vi "Assert Selection.vi"(9 "Actual":T1, 10 "Expected":T1, 11 "Added Section Finder Test In":refnum<class "Added Section Finder Test.lvclass">) -> (0 "error out":errorcluster, 3 "Added Section Finder Test Out":refnum<class "Added Section Finder Test.lvclass">)   [LabVIEW 2020, in "Added Section Finder Test.lvclass"]
uses:
  Added Section Finder Test.lvclass
  usr/local/natinst/LabVIEW-2026-64/vi.lib/Astemes/LUnit/Test Case.lvclass
  <vilib>/Astemes/LUnit/Test Case.lvclass/Test Case.ctl
  <vilib>/Astemes/LUnit/Test Case.lvclass
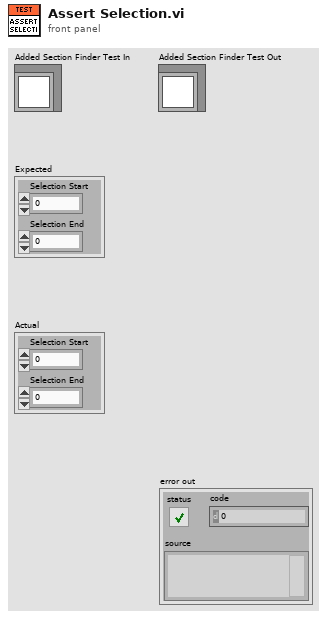
[diagram p1: front panel]
types:
  T1 = cluster{"Selection Start":u32, "Selection End":u32}
  T2 = cluster{"Selection Start":bool, "Selection End":bool}
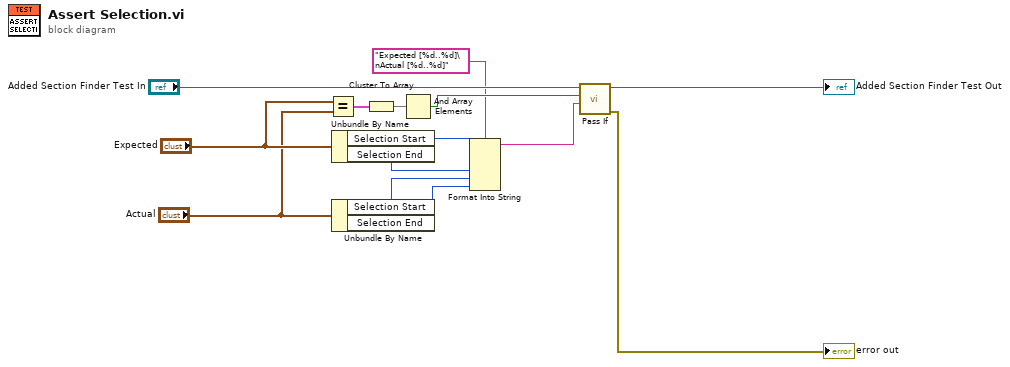
[diagram p0: block diagram]
diagram:
  n1 = Equal?(x="Expected", y="Actual") -> (x = y?=w9:T2)
  n2 = Unbundle By Name("Expected") -> ("Selection Start"=w5:u32, "Selection End"=w4:u32)
  n3 = Unbundle By Name("Actual") -> ("Selection Start"=w3:u32, "Selection End"=w2:u32)
  n4 = Cluster To Array(cluster=w9) -> (array=w8:bool[])
  n5 = And Array Elements(Boolean array=w8) -> (logical AND=w7:bool)
  n6 = Format Into String(format string="Expected [%d..%d]\nActual [%d..%d]", w5, w4, w3, w2) -> (resulting string=w1:string)  [unwired: 2 in, 1 out]
  n7 = call <vilib>:"Pass If.vi"("Message"=w1, "Pass?"=w7, "LUnit Test Case In"="Added Section Finder Test In") -> ("error out"=→"error out":errorcluster, "LUnit Test Case Out"=→"Added Section Finder Test Out":refnum<class "Added Section Finder Test.lvclass">)  [unwired: 7 in]
